vi "niRFUtil MT UTIL Filter Taps - Square Root Raised Cosine.vi"(0 "Samples Per Symbol (16)":i32=16, 5 "Filter Length (3)":i32=3, 7 "Alpha (0.5)":dbl=0.5 format="%.2f", 11 "error in (no error)":errorcluster) -> (4 "Filter Coefficients":T1 min=0 max=127 format="%.2f", 15 "error out":errorcluster)   [LabVIEW 2015, in "niRFUtil.lvlib"]
uses:
  niRFUtil.lvlib
  Includes/niRFUtil INC Real Array.ctl
panel:
  out "SRRC":sgl[](graph)
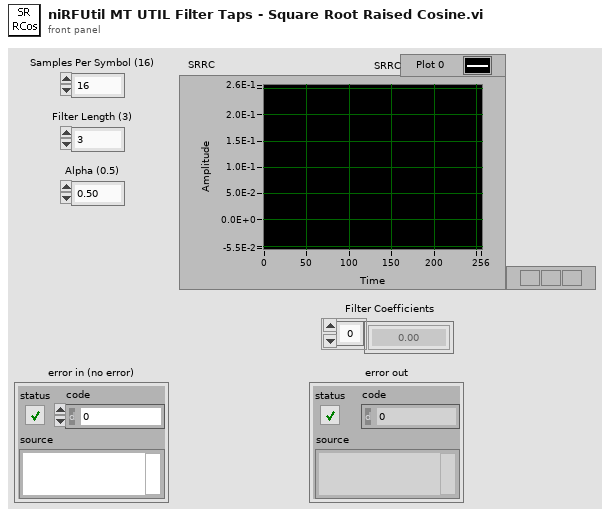
[diagram p1: front panel]
types:
  T1 = typedef "niRFUtil.lvlib/niRFUtil INC Real Array.ctl" = sgl[]
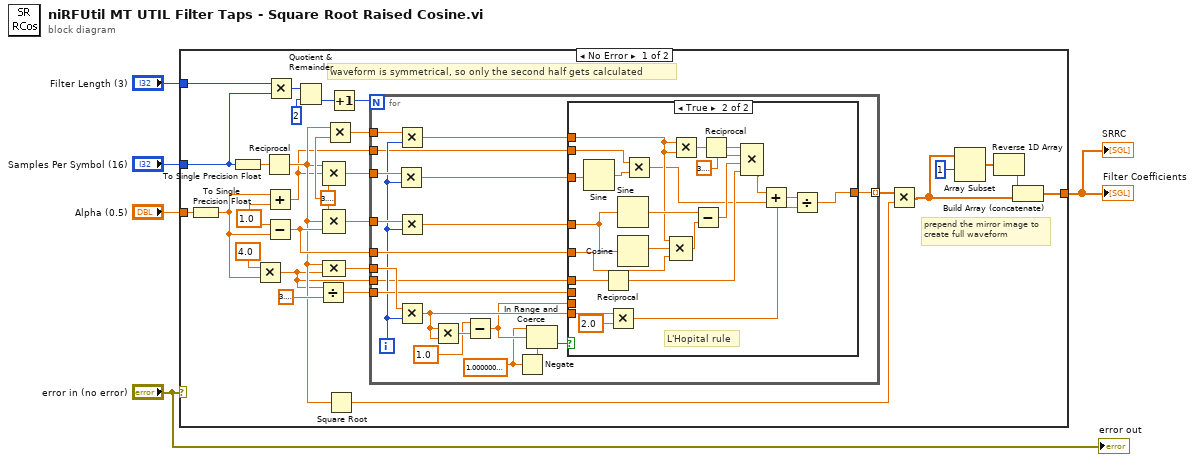
[diagram p0: block diagram]
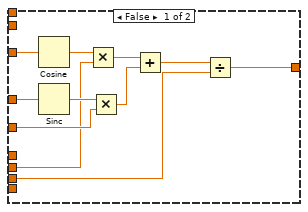
[diagram p2: hidden frame]
diagram:
  n1 = case shown="No Error" "error in (no error)" {
    tunnel: "Filter Length (3)" -> [w30 _]
    tunnel: "Samples Per Symbol (16)" -> [w8 _]
    tunnel: "Alpha (0.5)" -> [w7 _]
    tunnel: [w10 _] -> w2
    frame No Error {
      w28 = sgl 3.1415927
      w29 = sgl 1.0 ("y")
      # "waveform is symmetrical, so only the second half gets calculated"
      # "prepend the mirror image to create full waveform"
      n2 = To Single Precision Float(number=w7) -> (single precision float=w6:sgl)
      n3 = To Single Precision Float(number=w8) -> (single precision float=w9:sgl)
      n4 = Multiply(x=sgl 4.0 ("Input"), y=w6) -> (x*y=w12:sgl)
      n5 = Reciprocal(x=w9) -> (1/x=w14:sgl)
      n6 = Add(x=w6, y=w29) -> (x+y=w11:sgl)
      n7 = Subtract(x=w29, y=w6) -> (x-y=w23:sgl)
      n8 = Multiply(x=w30, y=w8) -> (x*y=w34:i32)
      n9 = Quotient & Remainder(x=w34, y=2) -> (floor(x/y)=w31:i32)  [unwired: 1 out]
      n10 = Divide(x=w12, y=sgl 3.1415927) -> (x/y=w21:sgl)
      n11 = Compound Arithmetic op=MULTIPLY(w14, w11, w28) -> (w27:sgl)
      n12 = Compound Arithmetic op=MULTIPLY(w28, w14, w23) -> (w26:sgl)
      n13 = Compound Arithmetic op=MULTIPLY(w14, w12) -> (w25:sgl)
      n14 = Multiply(x=w14, y=w28) -> (x*y=w13:sgl)
      n15 = Square Root(x=w14) -> (sqrt(x)=w19:sgl)
      n16 = Increment(x=w31) -> (x+1=w32:i32)
      n17 = for {
        N: w32 -> [_]
        tunnel: w27 -> [w52]
        tunnel: w26 -> [w53]
        tunnel: w25 -> [w54]
        tunnel: w23 -> [w47]
        tunnel: w21 -> [w46]
        tunnel: [w45] -> w20 mode=indexing
        tunnel: w13 -> [w44]
        tunnel: w12 -> [w41]
        tunnel: w11 -> [w40]
        i -> [w43]
        w36 = sgl 1e-07 ("y")
        n18 = Multiply(x=w52, y=w43) -> (x*y=w51:sgl)
        n19 = Multiply(x=w44, y=w43) -> (x*y=w42:sgl)
        n20 = Multiply(x=w53, y=w43) -> (x*y=w50:sgl)
        n21 = Multiply(x=w54, y=w43) -> (x*y=w39:sgl)
        n22 = Multiply(x=w39, y=w39) -> (x*y=w49:sgl)
        n23 = Subtract(x=sgl 1.0 ("y"), y=w49) -> (x-y=w37:sgl)
        n24 = Negate(x=w36) -> (-x=w35:sgl)
        n25 = In Range and Coerce(upper limit=w36, x=w37, lower limit=w35) -> (In Range?=w38:bool)  [unwired: 1 out]
        n26 = case shown="True" w38 {
          tunnel: w51 -> [w65 w76]
          tunnel: w50 -> [w64 w87]
          tunnel: w47 -> [w62 w66]
          tunnel: w46 -> [w60 _]
          tunnel: w37 -> [w56 _]
          tunnel: [w55 w67] -> w45
          tunnel: w42 -> [_ w83]
          tunnel: w41 -> [_ w79]
          tunnel: w40 -> [_ w74]
          tunnel: w39 -> [_ w70]
          frame False {
            n27 = Cosine(x=w65) -> (cos(x)=w61:sgl)
            n28 = Sinc(1:w64) -> (0:w63:sgl)
            n29 = Multiply(x=w61, y=w60) -> (x*y=w59:sgl)
            n30 = Multiply(x=w63, y=w62) -> (x*y=w58:sgl)
            n31 = Add(x=w59, y=w58) -> (x+y=w57:sgl)
            n32 = Divide(x=w57, y=w56) -> (x/y=w55:sgl)
          }
          frame True {
            # "L'Hopital rule"
            n33 = Sine(x=w76) -> (sin(x)=w75:sgl)
            n34 = Reciprocal(x=w79) -> (1/x=w78:sgl)
            n35 = Multiply(x=w70, y=sgl 2.0) -> (x*y=w68:sgl)
            n36 = Sine(x=w87) -> (sin(x)=w86:sgl)
            n37 = Cosine(x=w87) -> (cos(x)=w84:sgl)
            n38 = Multiply(x=w74, y=w75) -> (x*y=w72:sgl)
            n39 = Compound Arithmetic op=MULTIPLY(w83, w84, w66) -> (w85:sgl)
            n40 = Multiply(x=w83, y=w83) -> (x*y=w82:sgl)
            n41 = Subtract(x=w86, y=w85) -> (x-y=w77:sgl)
            n42 = Reciprocal(x=w82) -> (1/x=w81:sgl)
            n43 = Compound Arithmetic op=MULTIPLY(w81, sgl 3.1415927, w77, w78) -> (w73:sgl)
            n44 = Add(x=w73, y=w72) -> (x+y=w71:sgl)
            n45 = Divide(x=w71, y=w68) -> (x/y=w67:sgl)
          }
        }
      }
      n46 = Multiply(x=w20, y=w19) -> (x*y=w15:sgl[])
      n47 = Array Subset(array=w15, index=1 ("Array Index")) -> (w17:sgl[])  [unwired: 1 in]
      n48 = Reverse 1D Array(array=w17) -> (reversed array=w16:sgl[])
      n49 = Build Array (concatenate)(w16, w15) -> (w10:sgl[])
    }
    frame Error {
    }
  }
  "SRRC" <- w2
  "Filter Coefficients" <- w2
  "error out" <- "error in (no error)"
